vi "ReadDoubleGlobal.vi"(8 "error in (no error)":errorcluster, 9 "variable number":i32, 11 "controller in":refnum<k24>) -> (0 "error out":errorcluster, 2 "value":dbl, 3 "controller out":refnum<k24>)   [LabVIEW 2019]
uses:
  C:/Users/patrick/Documents/GitHub/Aerotech-Delay-Line/lvsrc/Aerotech-Ensemble-LabVIEW/2010-5.6/Bin/Aerotech.Ensemble.dll
  Bin/Aerotech.Ensemble.dll
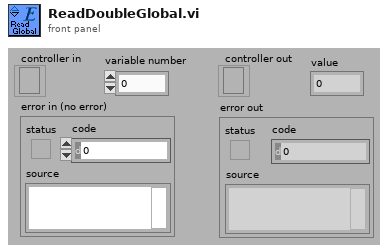
[diagram p1: front panel]
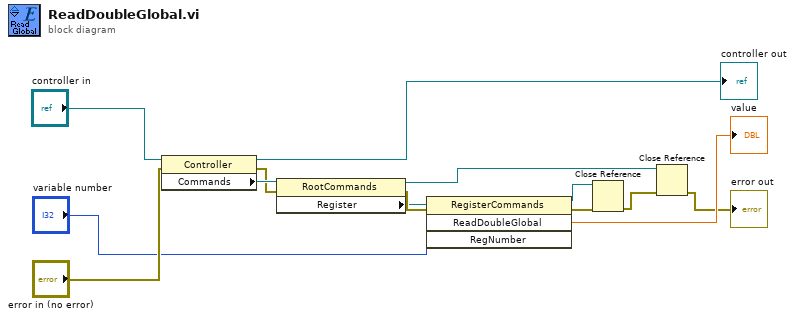
[diagram p0: block diagram]
diagram:
  n1 = property class="Controller"(reference="controller in", error in="error in (no error)") -> (reference out=→"controller out":refnum<k24>, error out=w10:errorcluster, "Commands"=w11:refnum<k24>)
  n2 = property class="RootCommands"(reference=w11, error in=w10) -> (reference out=w2:refnum<k24>, error out=w8:errorcluster, "Register"=w7:refnum<k24>)
  n3 = invoke class="RegisterCommands" method="ReadDoubleGlobal"(reference=w7, error in=w8, "RegNumber"="variable number") -> (reference out=w5:refnum<k24>, error out=w6:errorcluster, "ReadDoubleGlobal"=→"value":dbl)  [unwired: 1 in, 1 out]
  n4 = Close Reference(reference=w5, error in (no error)=w6) -> (error out=w4:errorcluster)
  n5 = Close Reference(reference=w2, error in (no error)=w4) -> (error out=→"error out":errorcluster)
